vi "Signals.SortByFrameLocation.vi"(8 "error in (no error)":errorcluster, 11 "Signals in":T1[](array[typedef]) {"Byte Order" items=["Little Endian", "Big Endian"]; "Data Type" items=["Signed", "Unsigned", "IEEE Float"]}) -> (0 "error out":errorcluster, 3 "Signals out":T1[](array[typedef]) {"Byte Order" items=["Little Endian", "Big Endian"]; "Data Type" items=["Signed", "Unsigned", "IEEE Float"]})   [LabVIEW 2019, in "Diagnostics Addon System Explorer.lvlib"]
uses:
  Diagnostics Addon System Explorer.lvlib
  Shared/Types/Signal.ctl
  Shared/SubVIs/Constants.vi
  <vilib>/xnet/xnet.llb/XNET Database Create (Cluster).vi
  <vilib>/xnet/xnet.llb/XNET Database Create (Frame).vi
  <vilib>/xnet/xnet.llb/XNET Database Create (Signal).vi
  <vilib>/xnet/xnet.llb/XNET Create Session (Conversion).vi
  <vilib>/xnet/xnet.llb/XNET Convert (Signal to Frame CAN).vi
  <vilib>/xnet/xnet.llb/XNET Database Delete (Cluster).vi
  <vilib>/xnet/xnet.llb/XNET Database Close (Database).vi
  <resource>/objmgr/xnet.rc
  Shared/Diagnostics Addon Shared.lvlib
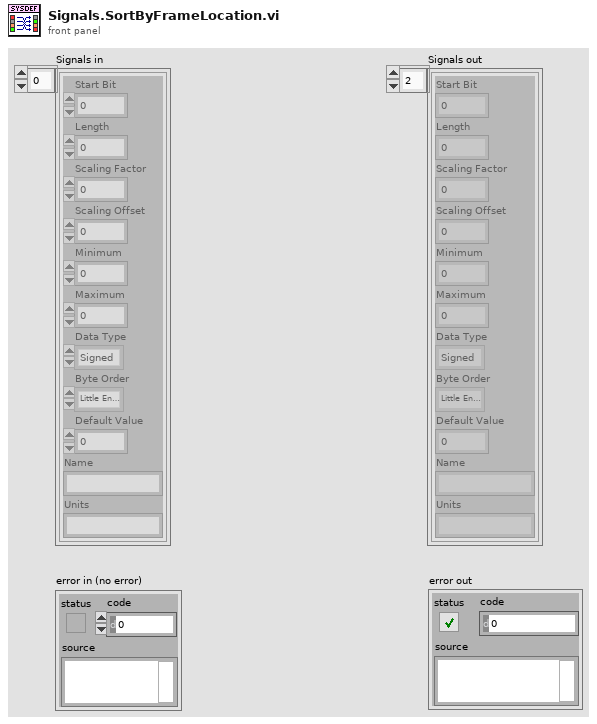
[diagram p1: front panel]
types:
  T1 = typedef "Diagnostics Addon Shared.lvlib/Signal.ctl" = cluster{"Start Bit":u32, "Length":u32, "Scaling Factor":dbl, "Scaling Offset":dbl, "Minimum":dbl, "Maximum":dbl, "Data Type":u32, "Byte Order":u32, "Default Value":dbl, "Name":string, "Units":string}
  T2 = typedef "XNET Frame CAN.ctl" = cluster{"timestamp":timestamp, "payload":u8[], "identifier":u32, "type":T3, "extended?":bool, "echo?":bool}
  T3 = typedef "XNET Frame Type CAN.ctl" = u8
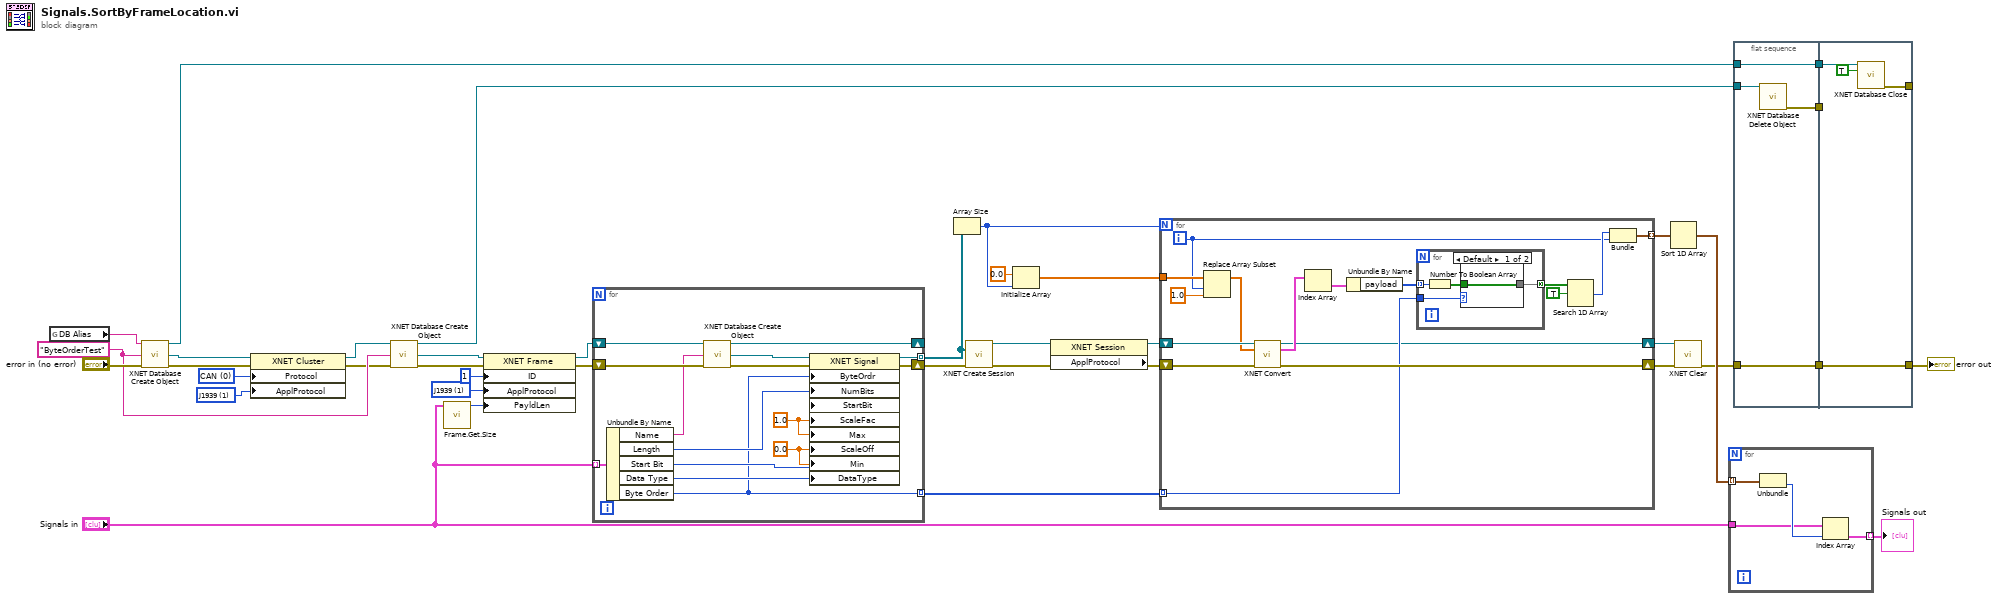
[diagram p0: block diagram]
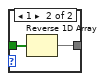
[diagram p2: hidden frame]
diagram:
  w2 = u32 1 items=["None", "J1939"] ("Application Protocol")
  w7 = u32 1 items=["None", "J1939"] ("Application Protocol")
  w8 = u32 0 items=["CAN", "FlexRay"] ("Protocol")
  w17 = "ByteOrderTest" ("frame name")
  n1 = global read "Constants.vi" "DB Alias"() -> (w18:string)
  n2 = call-poly <vilib>:"XNET Database Create Object.vi"("database in"=w18, "cluster name"=w17, "error in (no error)"="error in (no error)") -> ("database out"=w12:refnum<k21>, "cluster out"=w6:refnum<k21>, "error out"=w4:errorcluster)  [unwired: 10 in]
  n3 = property class="XNET Cluster"(reference=w6, error in=w4, "Protocol"=w8, "ApplProtocol"=w7) -> (reference out=w5:refnum<k21>, error out=w3:errorcluster)
  n4 = call-poly <vilib>:"XNET Database Create Object.vi"("cluster in"=w5, "frame name"=w17, "error in (no error)"=w3) -> ("cluster out"=w16:refnum<k21>, "frame out"=w32:refnum<k21>, "error out"=w31:errorcluster)  [unwired: 10 in]
  n5 = call "Frame.Get.Size.vi"("Parameters"="Signals in") -> ("Bytes"=w1:u32)  [unwired: 10 in]
  n6 = property class="XNET Frame"(reference=w32, error in=w31, "ID"=u32 1 ("Identifier"), "ApplProtocol"=w2, "PayldLen"=w1) -> (reference out=w30:refnum<k21>, error out=w29:errorcluster)
  n7 = for {
    tunnel: [w49] -> w20 mode=indexing
    shift-right: [w47] -> w34
    shift-left: w29 -> [w52]
    shift-right: [w46] -> _
    shift-left: w30 -> [w53]
    tunnel: "Signals in" -> [w45] mode=indexing
    tunnel: [w39] -> w27 mode=indexing
    w50 = 0.0 ("Scaling Offset")
    w40 = 1.0 ("Scaling Factor")
    n8 = Unbundle By Name(w45) -> ("Name"=w44:string, "Length"=w43:u32, "Start Bit"=w42:u32, "Data Type"=w41:u32, "Byte Order"=w39:u32)
    n9 = call-poly <vilib>:"XNET Database Create Object.vi"("frame in"=w53, "signal name"=w44, "error in (no error)"=w52) -> ("frame out"=w46:refnum<k21>, "signal out"=w51:refnum<k21>, "error out"=w48:errorcluster)  [unwired: 10 in]
    n10 = property class="XNET Signal"(reference=w51, error in=w48, "ByteOrdr"=w39, "NumBits"=w43, "StartBit"=w42, "ScaleFac"=w40, "Max"=w40, "ScaleOff"=w50, "Min"=w50, "DataType"=w41) -> (reference out=w49:refnum<k21>, error out=w47:errorcluster)
  }
  n11 = Array Size(array=w20) -> (size(s)=w35:i32)
  n12 = call-poly <vilib>:"XNET Create Session.vi"("signal list"=w20, "error in (no error)"=w34) -> ("session out"=w38:refnum<k21>, "error out"=w33:errorcluster)  [unwired: 12 in]
  n13 = Initialize Array(0.0 ("element"), w35) -> (w36:dbl[])
  n14 = property class="XNET Session" props=["ApplProtocol"](reference=w38) -> (reference out=w9:refnum<k21>)  [unwired: 1 in, 2 out]
  n15 = for {
    N: w35 -> [_]
    tunnel: w36 -> [w68]
    shift-right: [w65] -> w21
    shift-left: w33 -> [w66]
    tunnel: [w62] -> w28 mode=indexing
    tunnel: w27 -> [w56] mode=indexing
    shift-right: [w54] -> w22
    shift-left: w9 -> [w69]
    i -> [w55]
    n16 = Replace Array Subset(array=w68, new element=1.0 ("new element/subarray"), index=w55) -> (w57:dbl[])
    n17 = call-poly <vilib>:"XNET Convert.vi"("session in"=w69, "signal data"=w57, "error in (no error)"=w66) -> ("session out"=w54:refnum<k21>, "frame data"=w64:T2[], "error out"=w65:errorcluster)  [unwired: 9 in, 1 out]
    n18 = Index Array(array=w64) -> (element=w63:T2)  [unwired: 1 in]
    n19 = Unbundle By Name(w63) -> ("payload"=w61:u8[])
    n20 = for {
      tunnel: w61 -> [w73] mode=indexing
      tunnel: [w71] -> w60 mode=concatenating
      tunnel: w56 -> [w70]
      n21 = Number To Boolean Array(number=w73) -> (Boolean array=w72:bool[])
      n22 = case shown="Default" w70 {
        tunnel: w72 -> [w74 w76]
        tunnel: [w74 w75] -> w71
        frame Default {
        }
        frame 1 {
          n23 = Reverse 1D Array(array=w76) -> (reversed array=w75:bool[])
        }
      }
    }
    n24 = Search 1D Array(1D array=w60, element=TRUE) -> (index of element=w58:i32)  [unwired: 1 in]
    n25 = Bundle("index of element"=w58, w55) -> (w62:cluster{"index of element":i32, i32})  [unwired: 1 in]
  }
  n26 = Sort 1D Array(array=w28) -> (sorted array=w25:cluster{"index of element":i32, i32}[])
  n27 = call <vilib>:"XNET Clear.vi"("session in"=w22, "error in (no error)"=w21) -> ("error out"=w15:errorcluster)  [unwired: 13 in]
  n28 = for {
    tunnel: w25 -> [w80] mode=indexing
    tunnel: "Signals in" -> [w78]
    tunnel: [w77] -> w23 mode=indexing
    n29 = Unbundle(w80) -> (w79:i32)  [unwired: 1 out]
    n30 = Index Array(array=w78, index=w79) -> (element=w77:T1)
  }
  "Signals out" <- w23
  n31 = flat-sequence {
    tunnel: w16 -> [w84]
    tunnel: w15 -> [w81]
    tunnel: [w83] -> w14
    tunnel: [w82] -> w13
    tunnel: w12 -> [w82]
    tunnel: [w81] -> w10
    tunnel: w14 -> [_]
    tunnel: [w87] -> _
    tunnel: w13 -> [w86]
    tunnel: [w85] -> w11
    tunnel: w10 -> [w85]
    frame #0 {
      n32 = call-poly <vilib>:"XNET Database Delete Object.vi"("cluster in"=w84) -> ("error out"=w83:errorcluster)  [unwired: 14 in]
    }
    frame #1 {
      n33 = call-poly <vilib>:"XNET Database Close.vi"("database in"=w86, "close all? (true)"=TRUE) -> ("error out"=w87:errorcluster)  [unwired: 13 in]
    }
  }
  "error out" <- w11
